vi "Stop Point.vi"(7 "Point Ident":string, 8 "error in":errorcluster, 11 "MSS Target Actor in":refnum<class "MSS Target Actor.lvclass">) -> (0 "error out":errorcluster, 3 "MSS Target Actor out":refnum<class "MSS Target Actor.lvclass">)   [LabVIEW 2023, in "MSS Target Actor.lvlib" / "MSS Target Actor.lvclass"]
uses:
  MSS Target Actor.lvclass
  MSS Target Actor.lvclass/MSS Target Actor.ctl
  Measure and Stimulus Subsystems/Measure and Stimulus Subsystems.lvclass
  Study/Study Actor/IStudy Actor Messages/Log Target Msg/Log Target Msg.lvclass
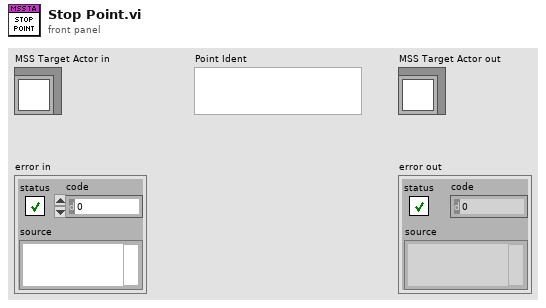
[diagram p1: front panel]
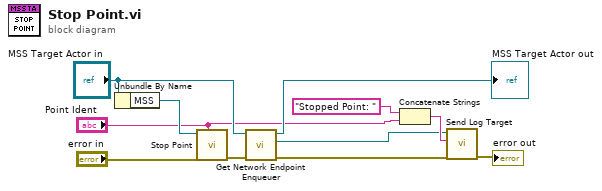
[diagram p0: block diagram]
diagram:
  n1 = Unbundle By Name("MSS Target Actor in") -> ("MSS"=w11:refnum<class "Measure and Stimulus Subsystems.lvclass">)
  n2 = call "Stop Point.vi"("Point Ident"="Point Ident", "error in"="error in", "MSS in"=w11) -> ("error out"=w9:errorcluster)  [unwired: 7 in, 1 out]
  n3 = call "Get Network Endpoint Enqueuer.vi"("error in"=w9, "MSS Target Actor in"="MSS Target Actor in") -> ("error out"=w1:errorcluster, "Enqueuer"=w2:refnum<class "Message Enqueuer.lvclass">, "MSS Target Actor out"=→"MSS Target Actor out":refnum<class "MSS Target Actor.lvclass">)  [unwired: 7 in]
  n4 = Concatenate Strings("Stopped Point: " ("string"), "Point Ident") -> (w3:string)
  n5 = call "Send Log Target.vi"("error in (no error)"=w1, "Entry"=w3, "Message Enqueuer"=w2) -> ("error out"=→"error out":errorcluster)  [unwired: 7 in, 1 out]
